vi "GetFloatFromNode(viaStringNodePath).vi"(2 "Path":string, 3 "error in":errorcluster, 5 "Tree DVR in":refnum<data-value>) -> (0 "error out":errorcluster, 1 "Float64":dbl)   [LabVIEW 2013]
uses:
  <vilib>/MDSplus/Classes/Tree_Class/Tree.lvclass
  <vilib>/MDSplus/Library/MDSplus.lvlib
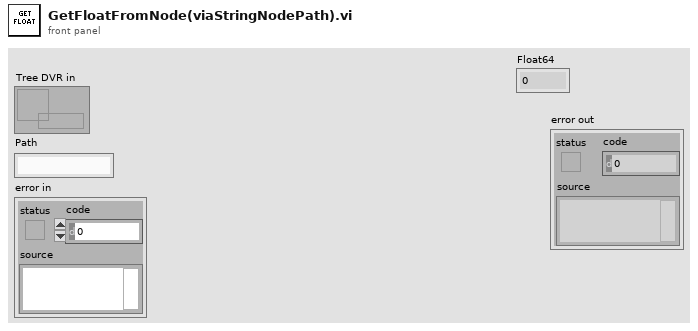
[diagram p1: front panel]
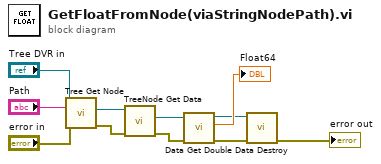
[diagram p0: block diagram]
diagram:
  n1 = call <vilib>:"Tree Get Node.vi"("error in (no error)"="error in", "Path"="Path", "Tree DVR in"="Tree DVR in") -> ("error out"=w10:errorcluster, "Node out"=w11:refnum<data-value>)  [unwired: 6 in, 1 out]
  n2 = call <vilib>:"TreeNode Get Data.vi"("error in (no error)"=w10, "TreeNode DVR in"=w11) -> ("error out"=w9:errorcluster, "Data out"=w8:refnum<data-value>)  [unwired: 7 in, 1 out]
  n3 = call <vilib>:"Data Get Double.vi"("error in (no error)"=w9, "Data DVR in"=w8) -> ("error out"=w2:errorcluster, "DBL out"=→"Float64":dbl, "Data DVR out"=w3:refnum<data-value>)  [unwired: 7 in]
  n4 = call <vilib>:"Data Destroy.vi"("error in (no error)"=w2, "Data DVR in"=w3) -> ("error out"=→"error out":errorcluster)  [unwired: 9 in]
